vi "Lab Panel V4.88.vi"() -> ()   [LabVIEW 2013] (continued)
              n212 = Bundle(cluster=w241, "Tmp Live"=w237, "Tmp Neut"=w236) -> (w239:T2)  [unwired: 3 in]
              n213 = local write "TEMP LA02"(w243) -> ()
              n214 = local write "SIG LAB02-1"(w239) -> ()
              n215 = local write "SIG LAB02-2"(w238) -> ()
            }
            frame #4 {
              w254 = 0
              n216 = local read "LAB03 TEMP"() -> (w256:T12)
              n217 = Unbundle By Name(w256) -> ("T1 Live"=w249:dbl, "T1 Neut"=w248:dbl, "T2 Live"=w247:dbl, "T2 Neut"=w246:dbl)  [unwired: 2 out]
              n218 = local read "SIG LAB03-1"() -> (w253:T2)
              n219 = local read "SIG LAB03-2"() -> (w252:T2)
              n220 = local read "TEMP LA03"() -> (w257:T9)
              n221 = Bundle By Name(cluster=w257, "TL-1"=w249, "TN-1"=w248, "TL-2"=w247, "TN-2"=w246, "TL -1COUNT"=w254, "TN-1 COUNT"=w254, "TL-2 COUNT"=w254, "TN-2 COUNT"=w254) -> (w255:T9)
              n222 = Bundle(cluster=w252, "Tmp Live"=w247, "Tmp Neut"=w246) -> (w250:T2)  [unwired: 3 in]
              n223 = Bundle(cluster=w253, "Tmp Live"=w249, "Tmp Neut"=w248) -> (w251:T2)  [unwired: 3 in]
              n224 = local write "TEMP LA03"(w255) -> ()
              n225 = local write "SIG LAB03-2"(w250) -> ()
              n226 = local write "SIG LAB03-1"(w251) -> ()
            }
            frame #5 {
              w266 = 0
              n227 = local read "LAB04 TEMP"() -> (w268:T12)
              n228 = Unbundle By Name(w268) -> ("T1 Live"=w261:dbl, "T1 Neut"=w260:dbl, "T2 Live"=w259:dbl, "T2 Neut"=w258:dbl)  [unwired: 2 out]
              n229 = local read "SIG LAB04-2"() -> (w264:T2)
              n230 = local read "SIG LAB04-1"() -> (w265:T2)
              n231 = local read "TEMP LA04"() -> (w269:T9)
              n232 = Bundle By Name(cluster=w269, "TL-1"=w261, "TN-1"=w260, "TL-2"=w259, "TN-2"=w258, "TL -1COUNT"=w266, "TN-1 COUNT"=w266, "TL-2 COUNT"=w266, "TN-2 COUNT"=w266) -> (w267:T9)
              n233 = Bundle(cluster=w264, "Tmp Live"=w259, "Tmp Neut"=w258) -> (w262:T2)  [unwired: 3 in]
              n234 = Bundle(cluster=w265, "Tmp Live"=w261, "Tmp Neut"=w260) -> (w263:T2)  [unwired: 3 in]
              n235 = local write "SIG LAB04-2"(w262) -> ()
              n236 = local write "TEMP LA04"(w267) -> ()
              n237 = local write "SIG LAB04-1"(w263) -> ()
            }
            frame #6 {
              w278 = 0
              n238 = local read "LAB05 TEMP"() -> (w280:T12)
              n239 = Unbundle By Name(w280) -> ("T1 Live"=w273:dbl, "T1 Neut"=w272:dbl, "T2 Live"=w271:dbl, "T2 Neut"=w270:dbl)  [unwired: 2 out]
              n240 = local read "SIG LAB05-2"() -> (w276:T2)
              n241 = local read "SIG LAB05-1"() -> (w277:T2)
              n242 = local read "TEMP LA05"() -> (w281:T9)
              n243 = Bundle By Name(cluster=w281, "TL-1"=w273, "TN-1"=w272, "TL-2"=w271, "TN-2"=w270, "TL -1COUNT"=w278, "TN-1 COUNT"=w278, "TL-2 COUNT"=w278, "TN-2 COUNT"=w278) -> (w279:T9)
              n244 = Bundle(cluster=w276, "Tmp Live"=w271, "Tmp Neut"=w270) -> (w274:T2)  [unwired: 3 in]
              n245 = Bundle(cluster=w277, "Tmp Live"=w273, "Tmp Neut"=w272) -> (w275:T2)  [unwired: 3 in]
              n246 = local write "SIG LAB05-2"(w274) -> ()
              n247 = local write "SIG LAB05-1"(w275) -> ()
              n248 = local write "TEMP LA05"(w279) -> ()
            }
          }
        }
        frame #8 {
          # "enable front panel, all settings done"
          n249 = property on="Tab Control 2" class="TabCtl (strict)"("DisabledEnum"=T16."Enabled" ("Disabled")) -> ()  [unwired: 2 in, 2 out]
          n250 = property on="Tab Control 2" class="TabCtl (strict)"("Value"=0) -> ()  [unwired: 2 in, 2 out]
        }
        frame #9 {
          n251 = property on="Tab Control 2" class="TabCtl (strict)"("Value"=0) -> ()  [unwired: 2 in, 2 out]
        }
      }
    }
    frame #2 {
      n252 = node-c288("loop  delay(mS)") -> (w287:T17)  [unwired: 3 in]
      n253 = timed-loop {
        timing: w287 -> [_]
        timing-out: [_] -> w286
        i -> [w309]
        stop <- "stop" stop-if-true
        n254 = node-c288() -> ()  [unwired: 1 in, 1 out]
        n255 = global write "Global display 1.vi" "stop disp"("stop") -> ()
        n256 = local read "SELECT LAB05-2"() -> (w289:T3)
        n257 = local read "SELECT LAB05-1"() -> (w290:T3)
        n258 = local read "SELECT LAB04-2"() -> (w291:T3)
        n259 = local read "SELECT LAB03-1"() -> (w294:T3)
        n260 = local read "SELECT LAB02-2"() -> (w295:T3)
        n261 = local read "SELECT LAB01-1"() -> (w298:T3)
        n262 = local read "SELECT LAB03-2"() -> (w293:T3)
        n263 = local read "SELECT LAB01-2"() -> (w297:T3)
        n264 = local read "SELECT LAB04-1"() -> (w292:T3)
        n265 = local read "SELECT LAB02-1"() -> (w296:T3)
        n266 = local read "run lab03-2"() -> (w303:bool)
        n267 = local read "run lab04-1"() -> (w302:bool)
        n268 = local read "run lab05-1"() -> (w300:bool)
        n269 = local read "run lab04-2"() -> (w301:bool)
        n270 = local read "run lab05-2"() -> (w299:bool)
        n271 = local read "run lab03-1"() -> (w304:bool)
        n272 = local read "run lab02-2"() -> (w305:bool)
        n273 = local read "run lab02-1"() -> (w306:bool)
        n274 = local read "run lab01-1"() -> (w308:bool)
        n275 = local read "run lab01-2"() -> (w307:bool)
        n276 = stacked-sequence {
          seq-local: [_ w374 _ _ _ _ _ _ _ _ _ _ _ _ _ _ _ _ _ _ _ _ _] -> [_ _ _ _ _ w2474 _ _ _ _ _ _ _ _ _ _ _ _ _ _ _ _ _]
          seq-local: [_ w373 _ _ _ _ _ _ _ _ _ _ _ _ _ _ _ _ _ _ _ _ _] -> [_ _ _ _ _ w2473 _ _ _ _ _ _ _ _ _ _ _ _ _ _ _ _ _]
          seq-local: [_ w360 _ _ _ _ _ _ _ _ _ _ _ _ _ _ _ _ _ _ _ _ _] -> [_ _ _ _ _ w2472 _ _ _ _ _ _ _ _ _ _ _ _ _ _ _ _ _]
          seq-local: [_ w359 _ _ _ _ _ _ _ _ _ _ _ _ _ _ _ _ _ _ _ _ _] -> [_ _ _ _ _ w2471 _ _ _ _ _ _ _ _ _ _ _ _ _ _ _ _ _]
          seq-local: [_ w358 _ _ _ _ _ _ _ _ _ _ _ _ _ _ _ _ _ _ _ _ _] -> [_ _ _ _ _ w2470 _ _ _ _ _ _ _ _ _ _ _ _ _ _ _ _ _]
          seq-local: [_ w357 _ _ _ _ _ _ _ _ _ _ _ _ _ _ _ _ _ _ _ _ _] -> [_ _ _ _ _ w2469 _ _ _ _ _ _ _ _ _ _ _ _ _ _ _ _ _]
          seq-local: [_ w356 _ _ _ _ _ _ _ _ _ _ _ _ _ _ _ _ _ _ _ _ _] -> [_ _ _ _ _ w2468 _ _ _ _ _ _ _ _ _ _ _ _ _ _ _ _ _]
          seq-local: [_ w355 _ _ _ _ _ _ _ _ _ _ _ _ _ _ _ _ _ _ _ _ _] -> [_ _ _ _ _ w2467 _ _ _ _ _ _ _ _ _ _ _ _ _ _ _ _ _]
          seq-local: [_ w354 _ _ _ _ _ _ _ _ _ _ _ _ _ _ _ _ _ _ _ _ _] -> [_ _ _ _ _ w2466 _ _ _ _ _ _ _ _ _ _ _ _ _ _ _ _ _]
          seq-local: [_ w353 _ _ _ _ _ _ _ _ _ _ _ _ _ _ _ _ _ _ _ _ _] -> [_ _ _ _ _ w2465 _ _ _ _ _ _ _ _ _ _ _ _ _ _ _ _ _]
          tunnel: w308 -> [_ _ w390 w637 w2064 w2494 w2809 w3296 _ _ _ _ w3721 _ w4678 _ _ w4965 w5268 w5450 _ _ _]
          tunnel: w307 -> [_ _ w389 w635 w2063 w2493 w2810 w3295 _ _ _ _ w3720 _ w4676 _ _ w4964 w5267 w5448 _ _ _]
          tunnel: w306 -> [_ _ w388 w633 w2062 w2492 w2808 w3294 _ _ _ _ w3719 _ w4674 _ _ w4963 w5266 w5447 _ _ _]
          tunnel: w305 -> [_ _ w387 w631 w2061 w2491 w2807 w3293 _ _ _ _ w3718 _ w4672 _ _ w4962 w5265 w5446 _ _ _]
          tunnel: w304 -> [_ _ w386 w629 w2060 w2490 w2806 w3292 _ _ _ _ w3717 _ w4670 _ _ w4961 w5264 w5445 _ _ _]
          tunnel: w303 -> [_ _ w385 w627 w2059 w2489 w2805 w3291 _ _ _ _ w3716 _ w4668 _ _ w4960 w5263 w5444 _ _ _]
          tunnel: w302 -> [_ _ w384 w625 w2058 w2488 w2804 w3290 _ _ _ _ w3715 _ w4666 _ _ w4959 w5262 w5443 _ _ _]
          tunnel: w301 -> [_ _ w383 w623 w2057 w2487 w2803 w3289 _ _ _ _ w3714 _ w4664 _ _ w4958 w5261 w5442 _ _ _]
          tunnel: w300 -> [_ _ w382 w621 w2056 w2486 w2802 w3288 _ _ _ _ w3713 _ w4662 _ _ w4957 w5260 w5441 _ _ _]
          tunnel: w299 -> [_ _ w381 w619 w2055 w2485 w2801 w3287 _ _ _ _ w3712 _ w4660 _ _ w4956 w5259 w5440 _ _ _]
          tunnel: w298 -> [_ _ _ w636 w2054 w2484 _ _ _ _ _ _ _ _ w4680 _ _ _ _ _ w5788 _ _]
          tunnel: w297 -> [_ _ _ w634 w2053 w2483 _ _ _ _ _ _ _ _ w4675 _ _ _ _ _ w5787 _ _]
          tunnel: w296 -> [_ _ _ w632 w2052 w2482 _ _ _ _ _ _ _ _ w4673 _ _ _ _ _ w5786 _ _]
          tunnel: w295 -> [_ _ _ w630 w2051 w2481 _ _ _ _ _ _ _ _ w4671 _ _ _ _ _ w5785 _ _]
          tunnel: w294 -> [_ _ _ w628 w2050 w2480 _ _ _ _ _ _ _ _ w4669 _ _ _ _ _ w5784 _ _]
          tunnel: w293 -> [_ _ _ w626 w2049 w2479 _ _ _ _ _ _ _ _ w4667 _ _ _ _ _ w5783 _ _]
          tunnel: w292 -> [_ _ _ w624 w2048 w2478 _ _ _ _ _ _ _ _ w4665 _ _ _ _ _ w5782 _ _]
          tunnel: w291 -> [_ _ _ w622 w2047 w2477 _ _ _ _ _ _ _ _ w4663 _ _ _ _ _ w5781 _ _]
          tunnel: w290 -> [_ _ _ w620 w2046 w2476 _ _ _ _ _ _ _ _ w4661 _ _ _ _ _ w5780 _ _]
          tunnel: w289 -> [_ _ _ w618 w2045 w2475 _ _ _ _ _ _ _ _ w4659 _ _ _ _ _ w5779 _ _]
          frame #0 {
            w316 = FALSE
            w321 = 0.5
            # "set up cycle control"
            n277 = local read "jig cycle"() -> (w320:dbl)
            n278 = local read "Amps Fail level"() -> (w314:dbl)
            n279 = Divide(x="JIG ON TIME (S)", y=w321) -> (x/y=→"on loops":dbl)
            n280 = Divide(x="JIG OFF TIME (S)", y=w321) -> (x/y=→"off loops":dbl)
            n281 = global write "Global display 3.vi" "Amps Fail"(w314) -> ()
            n282 = Increment(x=w320) -> (x+1=w319:dbl)
            n283 = local write "TEMP"(w316) -> ()
            n284 = local write "AI"(w316) -> ()
            n285 = local read "Network Directory"() -> (w313:path)
            n286 = local write "jig cycle"(w319) -> ()
            n287 = call "sub vi - check network dir v2.vi"("PATH"=w313) -> ("error"=w312:bool)  [unwired: 10 in]
            n288 = local write "network error"(w312) -> ()
            n289 = global write "Global display 3.vi" "network drive"(w312) -> ()
            n290 = event shown="[1] \"ADMIN\": Value Change" {
              selector: _ -> [_ _]
              dyn-events: _ -> [_ _]
              timeout: 10 -> [_ _]
              event Timeout {
                n291 = event-data() -> ()  [unwired: 1 in, 3 out]
              }
              event "ADMIN": Value Change {
                n292 = event-data() -> ()  [unwired: 1 in, 6 out]
                n293 = stacked-sequence {
                  seq-local: [_ w325 _] -> [_ _ w326]
                  frame #0 {
                    n294 = global write "Global 1.vi" "password"("9949") -> ()
                  }
                  frame #1 {
                    n295 = call "sub vi - password 1.vi"() -> ("RESULT"=w325:bool)  [unwired: 11 in]
                  }
                  frame #2 {
                    w328 = FALSE
                    n296 = property on="Tab Control 2" class="TabCtl (strict)"() -> ("Pages"=w332:refnum<vi>[])  [unwired: 2 in, 2 out]
                    n297 = Select(t=TRUE, s=w326, f=w328) -> (s? t:f=w327:bool)
                    n298 = Index Array(array=w332, index=8) -> (element=w330:refnum<vi>)
                    n299 = property class="Page"(reference=w330, "PageVis"=w327) -> ()  [unwired: 1 in, 2 out]
                    n300 = local write "ADMIN"(w328) -> ()
                  }
                }
              }
            }
          }
          frame #1 {
            w370 = 60.0
            # "convert temperature rise minutes to cycles"
            n301 = local read "SET LAB05-2"() -> (w334:T5)
            n302 = local read "SET LAB05-1"() -> (w336:T5)
            n303 = local read "SET LAB04-2"() -> (w338:T5)
            n304 = local read "SET LAB01-1"() -> (w352:T5)
            n305 = local read "SET LAB01-2"() -> (w350:T5)
            n306 = local read "SET LAB02-2"() -> (w346:T5)
            n307 = local read "SET LAB04-1"() -> (w340:T5)
            n308 = local read "SET LAB03-1"() -> (w344:T5)
            n309 = local read "SET LAB03-2"() -> (w342:T5)
            n310 = local read "SET LAB02-1"() -> (w348:T5)
            n311 = local read "JIG OFF TIME (S)"() -> (w375:dbl)
            n312 = local read "JIG ON TIME (S)"() -> (w376:dbl)
            n313 = Unbundle(w334) -> ("T-RISE mins"=w333:dbl)  [unwired: 4 out]
            n314 = Unbundle(w336) -> ("T-RISE mins"=w335:dbl)  [unwired: 4 out]
            n315 = Unbundle(w352) -> ("T-RISE mins"=w351:dbl)  [unwired: 4 out]
            n316 = Unbundle(w338) -> ("T-RISE mins"=w337:dbl)  [unwired: 4 out]
            n317 = Unbundle(w350) -> ("T-RISE mins"=w349:dbl)  [unwired: 4 out]
            n318 = Unbundle(w348) -> ("T-RISE mins"=w347:dbl)  [unwired: 4 out]
            n319 = Unbundle(w340) -> ("T-RISE mins"=w339:dbl)  [unwired: 4 out]
            n320 = Unbundle(w346) -> ("T-RISE mins"=w345:dbl)  [unwired: 4 out]
            n321 = Unbundle(w342) -> ("T-RISE mins"=w341:dbl)  [unwired: 4 out]
            n322 = Unbundle(w344) -> ("T-RISE mins"=w343:dbl)  [unwired: 4 out]
            n323 = Add(x=w376, y=w375) -> (x+y=w369:dbl)
            n324 = Multiply(x=w370, y=w341) -> (x*y=w365:dbl)
            n325 = Multiply(x=w370, y=w339) -> (x*y=w364:dbl)
            n326 = Multiply(x=w370, y=w337) -> (x*y=w363:dbl)
            n327 = Multiply(x=w370, y=w335) -> (x*y=w362:dbl)
            n328 = Multiply(x=w370, y=w333) -> (x*y=w361:dbl)
            n329 = Multiply(x=w370, y=w349) -> (x*y=w371:dbl)
            n330 = Multiply(x=w370, y=w343) -> (x*y=w366:dbl)
            n331 = Multiply(x=w370, y=w351) -> (x*y=w372:dbl)
            n332 = Multiply(x=w370, y=w347) -> (x*y=w368:dbl)
            n333 = Multiply(x=w370, y=w345) -> (x*y=w367:dbl)
            n334 = Divide(x=w362, y=w369) -> (x/y=w354:dbl)
            n335 = Divide(x=w363, y=w369) -> (x/y=w355:dbl)
            n336 = Divide(x=w364, y=w369) -> (x/y=w356:dbl)
            n337 = Divide(x=w361, y=w369) -> (x/y=w353:dbl)
            n338 = Divide(x=w366, y=w369) -> (x/y=w358:dbl)
            n339 = Divide(x=w372, y=w369) -> (x/y=w374:dbl)
            n340 = Divide(x=w371, y=w369) -> (x/y=w373:dbl)
            n341 = Divide(x=w368, y=w369) -> (x/y=w360:dbl)
            n342 = Divide(x=w367, y=w369) -> (x/y=w359:dbl)
            n343 = Divide(x=w365, y=w369) -> (x/y=w357:dbl)
          }
          frame #2 {
            # "control cycle loops"
            n344 = local read "JIG OFF TIME (S)"() -> (w379:dbl)
            n345 = local read "JIG ON TIME (S)"() -> (w378:dbl)
            n346 = local read "jig cycle"() -> (w392:dbl)
            n347 = local read "on loops"() -> (w394:dbl)
            n348 = local read "off loops"() -> (w393:dbl)
            n349 = Add(x=w379, y=w378) -> (x+y=w377:dbl)
            n350 = Add(x=w394, y=w393) -> (x+y=w380:dbl)
            n351 = Greater Or Equal?(x=w392, y=w380) -> (x >= y?=w391:bool)
            n352 = case shown="True" w391 {
              tunnel: w390 -> [_ w427]
              tunnel: w389 -> [_ w426]
              tunnel: w388 -> [_ w425]
              tunnel: w387 -> [_ w424]
              tunnel: w386 -> [_ w423]
              tunnel: w385 -> [_ w422]
              tunnel: w384 -> [_ w421]
              tunnel: w383 -> [_ w420]
              tunnel: w382 -> [_ w419]
              tunnel: w381 -> [_ w418]
              tunnel: w377 -> [_ w417]
              frame False {
              }
              frame True {
                # "increment cycle value and convert cycles to minutes for temp rise"
                n353 = stacked-sequence {
                  frame #0 {
                    n354 = local read "PANEL #"() -> (w430:dbl)
                    n355 = Increment(x=w430) -> (x+1=w429:dbl)
                    n356 = local write "PANEL #"(w429) -> ()
                  }
                  frame #1 {
                    n357 = local read "PANEL #"() -> (w431:dbl)
                    n358 = Greater?(x=w431, y=5) -> (0:w433:bool)
                    n359 = case shown="True" w433 {
                      frame False {
                      }
                      frame True {
                        n360 = local write "PANEL #"(1) -> ()
                      }
                    }
                  }
                }
                n361 = local read "JIG RELAY CYCLES"() -> (w416:T8)
                n362 = Unbundle By Name(w416) -> ("LAB01-1"=w414:dbl, "LAB01-2"=w412:dbl, "LAB02-1"=w410:dbl, "LAB02-2"=w408:dbl, "LAB03-1"=w406:dbl, "LAB03-2"=w404:dbl, "LAB04-1"=w402:dbl, "LAB04-2"=w400:dbl, "LAB05-1"=w398:dbl, "LAB05-2"=w396:dbl)
                n363 = stacked-sequence {
                  tunnel: w427 -> [w445 _ _ _ _ _ _ _ _ _]
                  tunnel: w426 -> [_ w462 _ _ _ _ _ _ _ _]
                  tunnel: w425 -> [_ _ w479 _ _ _ _ _ _ _]
                  tunnel: w424 -> [_ _ _ w496 _ _ _ _ _ _]
                  tunnel: w423 -> [_ _ _ _ w513 _ _ _ _ _]
                  tunnel: w422 -> [_ _ _ _ _ w530 _ _ _ _]
                  tunnel: w421 -> [_ _ _ _ _ _ w547 _ _ _]
                  tunnel: w420 -> [_ _ _ _ _ _ _ w564 _ _]
                  tunnel: w419 -> [_ _ _ _ _ _ _ _ w581 _]
                  tunnel: w418 -> [_ _ _ _ _ _ _ _ _ w598]
                  tunnel: w417 -> [w442 w459 w476 w493 w510 w527 w544 w561 w578 w595]
                  tunnel: w414 -> [w436 _ _ _ _ _ _ _ _ _]
                  tunnel: [w435 _ _ _ _ _ _ _ _ _] -> w413
                  tunnel: w412 -> [_ w453 _ _ _ _ _ _ _ _]
                  tunnel: [_ w452 _ _ _ _ _ _ _ _] -> w411
                  tunnel: w410 -> [_ _ w470 _ _ _ _ _ _ _]
                  tunnel: [_ _ w469 _ _ _ _ _ _ _] -> w409
                  tunnel: w408 -> [_ _ _ w487 _ _ _ _ _ _]
                  tunnel: [_ _ _ w486 _ _ _ _ _ _] -> w407
                  tunnel: w406 -> [_ _ _ _ w504 _ _ _ _ _]
                  tunnel: [_ _ _ _ w503 _ _ _ _ _] -> w405
                  tunnel: w404 -> [_ _ _ _ _ w521 _ _ _ _]
                  tunnel: [_ _ _ _ _ w520 _ _ _ _] -> w403
                  tunnel: w402 -> [_ _ _ _ _ _ w538 _ _ _]
                  tunnel: [_ _ _ _ _ _ w537 _ _ _] -> w401
                  tunnel: w400 -> [_ _ _ _ _ _ _ w555 _ _]
                  tunnel: [_ _ _ _ _ _ _ w554 _ _] -> w399
                  tunnel: w398 -> [_ _ _ _ _ _ _ _ w572 _]
                  tunnel: [_ _ _ _ _ _ _ _ w571 _] -> w397
                  tunnel: w396 -> [_ _ _ _ _ _ _ _ _ w589]
                  tunnel: [_ _ _ _ _ _ _ _ _ w588] -> w395
                  frame #0 {
                    n364 = local read "DISP LAB01-1"() -> (w440:T4)
                    n365 = Unbundle(w440) -> ("CYCLE"=w441:dbl)  [unwired: 2 out]
                    n366 = case shown="True" w445 {
                      tunnel: w441 -> [w447 w451]
                      tunnel: [w447 w450] -> w439
                      tunnel: w436 -> [w446 w449]
                      tunnel: [w446 w448] -> w435
                      frame False {
                      }
                      frame True {
                        n367 = Increment(x=w449) -> (x+1=w448:dbl)
                        n368 = Increment(x=w451) -> (x+1=w450:dbl)
                      }
                    }
                    n369 = Multiply(x=w439, y=w442) -> (x*y=w443:dbl)
                    n370 = Divide(x=w443, y=60.0) -> (x/y=w438:dbl)
                    n371 = Bundle(cluster=w440, "CYCLE"=w439, "MINS"=w438) -> (w437:T4)  [unwired: 1 in]
                    n372 = local write "DISP LAB01-1"(w437) -> ()
                  }
                  frame #1 {
                    n373 = local read "DISP LAB01-2"() -> (w457:T4)
                    n374 = Unbundle(w457) -> ("CYCLE"=w458:dbl)  [unwired: 2 out]
                    n375 = case shown="True" w462 {
                      tunnel: w458 -> [w464 w468]
                      tunnel: [w464 w467] -> w455
                      tunnel: w453 -> [w463 w466]
                      tunnel: [w463 w465] -> w452
                      frame False {
                      }
                      frame True {
                        n376 = Increment(x=w466) -> (x+1=w465:dbl)
                        n377 = Increment(x=w468) -> (x+1=w467:dbl)
                      }
                    }
                    n378 = Multiply(x=w455, y=w459) -> (x*y=w460:dbl)
                    n379 = Divide(x=w460, y=60.0) -> (x/y=w454:dbl)
                    n380 = Bundle(cluster=w457, "CYCLE"=w455, "MINS"=w454) -> (w456:T4)  [unwired: 1 in]
                    n381 = local write "DISP LAB01-2"(w456) -> ()
                  }
                  frame #2 {
                    n382 = local read "DISP LAB02-1"() -> (w474:T4)
                    n383 = Unbundle(w474) -> ("CYCLE"=w475:dbl)  [unwired: 2 out]
                    n384 = case shown="True" w479 {
                      tunnel: [w481 w485] -> w472
                      tunnel: w475 -> [w481 w484]
                      tunnel: w470 -> [w480 w483]
                      tunnel: [w480 w482] -> w469
                      frame False {
                      }
                      frame True {
                        n385 = Increment(x=w483) -> (x+1=w482:dbl)
                        n386 = Increment(x=w484) -> (x+1=w485:dbl)
                      }
                    }
                    n387 = Multiply(x=w472, y=w476) -> (x*y=w477:dbl)
                    n388 = Divide(x=w477, y=60.0) -> (x/y=w471:dbl)
                    n389 = Bundle(cluster=w474, "CYCLE"=w472, "MINS"=w471) -> (w473:T4)  [unwired: 1 in]
                    n390 = local write "DISP LAB02-1"(w473) -> ()
                  }
                  frame #3 {
                    n391 = local read "DISP LAB02-2"() -> (w491:T4)
                    n392 = Unbundle(w491) -> ("CYCLE"=w492:dbl)  [unwired: 2 out]
                    n393 = case shown="True" w496 {
                      tunnel: [w498 w502] -> w490
                      tunnel: w492 -> [w498 w501]
                      tunnel: w487 -> [w497 w500]
                      tunnel: [w497 w499] -> w486
                      frame False {
                      }
                      frame True {
                        n394 = Increment(x=w500) -> (x+1=w499:dbl)
                        n395 = Increment(x=w501) -> (x+1=w502:dbl)
                      }
                    }
                    n396 = Multiply(x=w490, y=w493) -> (x*y=w494:dbl)
                    n397 = Divide(x=w494, y=60.0) -> (x/y=w489:dbl)
                    n398 = Bundle(cluster=w491, "CYCLE"=w490, "MINS"=w489) -> (w488:T4)  [unwired: 1 in]
                    n399 = local write "DISP LAB02-2"(w488) -> ()
                  }
                  frame #4 {
                    n400 = local read "DISP LAB03-1"() -> (w508:T4)
                    n401 = Unbundle(w508) -> ("CYCLE"=w509:dbl)  [unwired: 2 out]
                    n402 = case shown="True" w513 {
                      tunnel: [w515 w519] -> w505
                      tunnel: w509 -> [w515 w518]
                      tunnel: w504 -> [w514 w517]
                      tunnel: [w514 w516] -> w503
                      frame False {
                      }
                      frame True {
                        n403 = Increment(x=w517) -> (x+1=w516:dbl)
                        n404 = Increment(x=w518) -> (x+1=w519:dbl)
                      }
                    }
                    n405 = Multiply(x=w505, y=w510) -> (x*y=w511:dbl)
                    n406 = Divide(x=w511, y=60.0) -> (x/y=w506:dbl)
                    n407 = Bundle(cluster=w508, "CYCLE"=w505, "MINS"=w506) -> (w507:T4)  [unwired: 1 in]
                    n408 = local write "DISP LAB03-1"(w507) -> ()
                  }
                  frame #5 {
                    n409 = local read "DISP LAB03-2"() -> (w525:T4)
                    n410 = Unbundle(w525) -> ("CYCLE"=w526:dbl)  [unwired: 2 out]
                    n411 = case shown="True" w530 {
                      tunnel: [w532 w536] -> w524
                      tunnel: w526 -> [w532 w535]
                      tunnel: w521 -> [w531 w534]
                      tunnel: [w531 w533] -> w520
                      frame False {
                      }
                      frame True {
                        n412 = Increment(x=w534) -> (x+1=w533:dbl)
                        n413 = Increment(x=w535) -> (x+1=w536:dbl)
                      }
                    }
                    n414 = Multiply(x=w524, y=w527) -> (x*y=w528:dbl)
                    n415 = Divide(x=w528, y=60.0) -> (x/y=w523:dbl)
                    n416 = Bundle(cluster=w525, "CYCLE"=w524, "MINS"=w523) -> (w522:T4)  [unwired: 1 in]
                    n417 = local write "DISP LAB03-2"(w522) -> ()
                  }
                  frame #6 {
                    n418 = local read "DISP LAB04-1"() -> (w542:T4)
                    n419 = Unbundle(w542) -> ("CYCLE"=w543:dbl)  [unwired: 2 out]
                    n420 = case shown="True" w547 {
                      tunnel: [w549 w553] -> w540
                      tunnel: w543 -> [w549 w552]
                      tunnel: w538 -> [w548 w551]
                      tunnel: [w548 w550] -> w537
                      frame False {
                      }
                      frame True {
                        n421 = Increment(x=w551) -> (x+1=w550:dbl)
                        n422 = Increment(x=w552) -> (x+1=w553:dbl)
                      }
                    }
                    n423 = Multiply(x=w540, y=w544) -> (x*y=w545:dbl)
                    n424 = Divide(x=w545, y=60.0) -> (x/y=w539:dbl)
                    n425 = Bundle(cluster=w542, "CYCLE"=w540, "MINS"=w539) -> (w541:T4)  [unwired: 1 in]
                    n426 = local write "DISP LAB04-1"(w541) -> ()
                  }
                  frame #7 {
                    n427 = local read "DISP LAB04-2"() -> (w559:T4)
                    n428 = Unbundle(w559) -> ("CYCLE"=w560:dbl)  [unwired: 2 out]
                    n429 = case shown="True" w564 {
                      tunnel: [w566 w570] -> w557
                      tunnel: w560 -> [w566 w569]
                      tunnel: w555 -> [w565 w568]
                      tunnel: [w565 w567] -> w554
                      frame False {
                      }
                      frame True {
                        n430 = Increment(x=w568) -> (x+1=w567:dbl)
                        n431 = Increment(x=w569) -> (x+1=w570:dbl)
                      }
                    }
                    n432 = Multiply(x=w557, y=w561) -> (x*y=w563:dbl)
                    n433 = Divide(x=w563, y=60.0) -> (x/y=w556:dbl)
                    n434 = Bundle(cluster=w559, "CYCLE"=w557, "MINS"=w556) -> (w558:T4)  [unwired: 1 in]
                    n435 = local write "DISP LAB04-2"(w558) -> ()
                  }
                  frame #8 {
                    n436 = local read "DISP LAB05-1"() -> (w576:T4)
                    n437 = Unbundle(w576) -> ("CYCLE"=w577:dbl)  [unwired: 2 out]
                    n438 = case shown="True" w581 {
                      tunnel: [w583 w587] -> w574
                      tunnel: w577 -> [w583 w586]
                      tunnel: w572 -> [w582 w585]
                      tunnel: [w582 w584] -> w571
                      frame False {
                      }
                      frame True {
                        n439 = Increment(x=w585) -> (x+1=w584:dbl)
                        n440 = Increment(x=w586) -> (x+1=w587:dbl)
                      }
                    }
                    n441 = Multiply(x=w574, y=w578) -> (x*y=w579:dbl)
                    n442 = Divide(x=w579, y=60.0) -> (x/y=w573:dbl)
                    n443 = Bundle(cluster=w576, "CYCLE"=w574, "MINS"=w573) -> (w575:T4)  [unwired: 1 in]
                    n444 = local write "DISP LAB05-1"(w575) -> ()
                  }
                  frame #9 {
                    n445 = local read "DISP LAB05-2"() -> (w594:T4)
                    n446 = Unbundle(w594) -> ("CYCLE"=w593:dbl)  [unwired: 2 out]
                    n447 = case shown="True" w598 {
                      tunnel: [w600 w604] -> w592
                      tunnel: w593 -> [w600 w603]
                      tunnel: w589 -> [w599 w602]
                      tunnel: [w599 w601] -> w588
                      frame False {
                      }
                      frame True {
                        n448 = Increment(x=w602) -> (x+1=w601:dbl)
                        n449 = Increment(x=w603) -> (x+1=w604:dbl)
                      }
                    }
                    n450 = Multiply(x=w592, y=w595) -> (x*y=w596:dbl)
                    n451 = Divide(x=w596, y=60.0) -> (x/y=w591:dbl)
                    n452 = Bundle(cluster=w594, "CYCLE"=w592, "MINS"=w591) -> (w590:T4)  [unwired: 1 in]
                    n453 = local write "DISP LAB05-2"(w590) -> ()
                  }
                }
                n454 = local write "jig cycle"(0) -> ()
                n455 = Bundle By Name(cluster=w416, "LAB01-1"=w413, "LAB01-2"=w411, "LAB02-1"=w409, "LAB02-2"=w407, "LAB03-1"=w405, "LAB03-2"=w403, "LAB04-1"=w401, "LAB04-2"=w399, "LAB05-1"=w397, "LAB05-2"=w395) -> (w415:T8)
                n456 = local write "JIG RELAY CYCLES"(w415) -> ()
              }
            }
          }
          frame #3 {
            # "START & STOP test RUN switch change, start test if true and stop test if false"
            n457 = Get Date/Time In Seconds() -> (seconds since 1Jan1904=w616:timestamp)
            n458 = local read "C drive data root dir"() -> (w609:path)
            n459 = Format Date/Time String(time format string (%c)="%b\\%a%d", seconds (now)=w616) -> (date/time string=w640:string)  [unwired: 1 in]
            n460 = Format Date/Time String(time format string (%c)="%H%M", seconds (now)=w616) -> (date/time string=w638:string)  [unwired: 1 in]
            n461 = Format Date/Time String(time format string (%c)="LabPanel%Y", seconds (now)=w616) -> (date/time string=w615:string)  [unwired: 1 in]
            n462 = Path To String(path=w609) -> (string=w612:string)
            n463 = global write "Global 1.vi" "C drive root path"(w609) -> ()
            n464 = local read "Ref deg C"() -> (w605:dbl)
            n465 = Concatenate Strings(w612, "\\") -> (w610:string)
            n466 = event shown="[1] \"RUN LAB01-1\": Value Change" {
              selector: _ -> [_ _ _ _ _ _ _ _ _ _ _]
              dyn-events: _ -> [_ _ _ _ _ _ _ _ _ _ _]
              timeout: 10 -> [_ _ _ _ _ _ _ _ _ _ _]
              tunnel: w610 -> [_ w653 w793 w934 w1074 w1214 w1354 w1494 w1634 w1774 w1915]
              tunnel: w640 -> [_ w652 w792 w933 w1073 w1213 w1353 w1493 w1633 w1773 w1914]
              tunnel: w638 -> [_ w650 w791 w932 w1072 w1212 w1352 w1492 w1632 w1772 w1913]
              tunnel: w636 -> [_ w651 _ _ _ _ _ _ _ _ _]
              tunnel: w637 -> [_ _ _ _ _ _ _ _ _ _ _]
              tunnel: w635 -> [_ _ _ _ _ _ _ _ _ _ _]
              tunnel: w634 -> [_ _ w790 _ _ _ _ _ _ _ _]
              tunnel: w633 -> [_ _ _ _ _ _ _ _ _ _ _]
              tunnel: w632 -> [_ _ _ w931 _ _ _ _ _ _ _]
              tunnel: w631 -> [_ _ _ _ _ _ _ _ _ _ _]
              tunnel: w630 -> [_ _ _ _ w1071 _ _ _ _ _ _]
              tunnel: w629 -> [_ _ _ _ _ _ _ _ _ _ _]
              tunnel: w628 -> [_ _ _ _ _ w1211 _ _ _ _ _]
              tunnel: w627 -> [_ _ _ _ _ _ _ _ _ _ _]
              tunnel: w626 -> [_ _ _ _ _ _ w1351 _ _ _ _]
              tunnel: w625 -> [_ _ _ _ _ _ _ _ _ _ _]
              tunnel: w624 -> [_ _ _ _ _ _ _ w1491 _ _ _]
              tunnel: w623 -> [_ _ _ _ _ _ _ _ _ _ _]
              tunnel: w622 -> [_ _ _ _ _ _ _ _ w1631 _ _]
              tunnel: w621 -> [_ _ _ _ _ _ _ _ _ _ _]
              tunnel: w620 -> [_ _ _ _ _ _ _ _ _ w1771 _]
              tunnel: w619 -> [_ _ _ _ _ _ _ _ _ _ _]
              tunnel: w618 -> [_ _ _ _ _ _ _ _ _ _ w1912]
              tunnel: w615 -> [_ w649 w789 w930 w1070 w1210 w1350 w1490 w1630 w1770 w1911]
              tunnel: [_ w648 w788 w929 w1069 w1209 w1349 w1489 w1629 w1769 w1910] -> w613
              tunnel: "RESET CYCLES TO ZERO?" -> [_ w647 w786 w927 w1067 w1207 w1347 w1487 w1627 w1767 w1908]
              tunnel: "YES" -> [_ w646 w785 w926 w1066 w1206 w1346 w1486 w1626 w1766 w1907]
              tunnel: "NO" -> [_ w645 w784 w925 w1065 w1205 w1345 w1485 w1625 w1765 w1906]
              tunnel: w605 -> [_ w642 w783 w923 w1064 w1204 w1344 w1484 w1624 w1764 w1904]
              event Timeout {
                n467 = event-data() -> ()  [unwired: 1 in, 3 out]
              }
              event "RUN LAB01-1": Value Change {
                n468 = event-data() -> ("NewVal"=w643:bool)  [unwired: 1 in, 5 out]
                n469 = local read "SIG LAB01-1"() -> (w644:T2)
                n470 = local write "run lab01-1"(w643) -> ()
                n471 = case shown="True" w643 {
                  tunnel: w653 -> [_ w691]
                  tunnel: w652 -> [_ w690]
                  tunnel: w651 -> [w655 w689]
                  tunnel: w650 -> [_ w688]
                  tunnel: w649 -> [_ w687]
                  tunnel: [w654 w686] -> w648
                  tunnel: w647 -> [_ w685]
                  tunnel: w646 -> [_ w684]
                  tunnel: w645 -> [_ w683]
                  tunnel: w644 -> [_ w682]
                  tunnel: w642 -> [_ w681]
                  frame False {
                    # "stop test"
                    n472 = stacked-sequence {
                      tunnel: w655 -> [_ w667 _]
                      tunnel: [_ w659 _] -> w654
                      frame #0 {
                        n473 = local read "DISP LAB01-1"() -> (w658:T4)
                        n474 = Bundle(cluster=w658, "STATUS"="STOP") -> (w656:T4)  [unwired: 2 in]
                        n475 = local write "DISP LAB01-1"(w656) -> ()
                      }
                      frame #1 {
                        n476 = local read "DISP LAB01-1"() -> (w666:T4)
                        n477 = Unbundle(w666) -> ("CYCLE"=w664:dbl, "MINS"=w665:dbl)  [unwired: 1 out]
                        n478 = case shown="\"CYCLE TEST\"" w667 {
                          tunnel: w665 -> [_ _ w674]
                          tunnel: w664 -> [w672 w673 _]
                          tunnel: [w672 w673 w674] -> w663
                          frame "CHART TEST", Default {
                          }
                          frame "CYCLE TEST" {
                          }
                          frame "T-RISE TEST" {
                          }
                        }
                        n479 = local read "TDMS LAB01-1"() -> (w671:refnum<k34>)
                        n480 = Build Array("STOPPED") -> (w668:string[])
                        n481 = Build Array(w663) -> (w662:dbl[])
                        n482 = TDMS Write(0:w671, 5:"TEST RESULT", 7:w668, 9:w662) -> (4:w660:refnum<k34>, 15:w661:errorcluster)  [unwired: 2 in, 2 out]
                        n483 = TDMS Close(8:w661, 11:w660) -> (0:w659:errorcluster)  [unwired: 1 out]
                      }
                      frame #2 {
                        n484 = stacked-sequence {
                          tunnel: "LAB01-1" -> [w677 w679]
                          frame #0 {
                            n485 = call "sub vi - defrag tdms v1.vi"("panel id"=w677) -> ("error out"=w676:errorcluster)  [unwired: 10 in]
                            n486 = local write "data file error"(w676) -> ()
                          }
                          frame #1 {
                            n487 = call "Save data file (stop) v3.vi"("panel id"=w679) -> ("network file save error"=w678:errorcluster)  [unwired: 9 in, 1 out]
                            n488 = local write "RESULT LAB01-1"(FALSE) -> ()
                            n489 = local write "data file error"(w678) -> ()
                          }
                        }
                      }
                    }
                  }
                  frame True {
                    n490 = stacked-sequence {
                      seq-local: [w693 _] -> [_ w697]
                      tunnel: w691 -> [_ w707]
                      tunnel: w690 -> [_ w706]
                      tunnel: w689 -> [_ w705]
                      tunnel: w688 -> [_ w704]
                      tunnel: w687 -> [_ w703]
                      tunnel: [_ w702] -> w686
                      tunnel: w685 -> [_ w701]
                      tunnel: w684 -> [_ w700]
                      tunnel: w683 -> [_ w699]
                      tunnel: w682 -> [w695 w698]
                      tunnel: w681 -> [_ w696]
                      frame #0 {
                        n491 = Unbundle(w695) -> ("AMPS"=w694:dbl)  [unwired: 4 out]
                        n492 = call "Check For Amps on v1.vi"("ID"="LAB01-1", "amps"=w694) -> ("amps"=w693:bool)  [unwired: 9 in]
                      }
                      frame #1 {
                        n493 = case shown="True" w697 {
                          tunnel: w707 -> [_ w720]
                          tunnel: w706 -> [_ w719]
                          tunnel: w705 -> [_ w718]
                          tunnel: w704 -> [_ w717]
                          tunnel: w703 -> [_ w716]
                          tunnel: [errorcluster {"status"=FALSE, "code"=0, "source"=""} ("error out") w715] -> w702
                          tunnel: w701 -> [_ w714]
                          tunnel: w700 -> [_ w713]
                          tunnel: w699 -> [_ w712]
                          tunnel: w698 -> [_ w711]
                          tunnel: w696 -> [_ w710]
                          frame False {
                            w708 = FALSE
                            n494 = local write "RUN LAB01-1"(w708) -> ()
                            n495 = local write "run lab01-1"(w708) -> ()
                          }
                          frame True {
                            n496 = stacked-sequence {
                              seq-local: [w721 _ _ _ _] -> [_ w742 _ _ _]
                              tunnel: w720 -> [w726 _ _ _ _]
                              tunnel: w719 -> [w722 _ _ _ _]
                              tunnel: w718 -> [w736 _ _ _ _]
                              tunnel: w717 -> [w729 _ _ _ _]
                              tunnel: w716 -> [w724 _ _ _ _]
                              tunnel: [_ w743 _ _ _] -> w715
                              tunnel: w714 -> [_ _ _ w764 _]
                              tunnel: w713 -> [_ _ _ w774 _]
                              tunnel: w712 -> [_ _ _ w773 _]
                              tunnel: w711 -> [_ _ _ _ _]
                              tunnel: w710 -> [_ _ _ _ w780]
                              frame #0 {
                                w723 = "\\"
                                n497 = case shown="\"CHART TEST\", Default" w736 {
                                tunnel: ["L01-1-CHART TEST-" "L01-1-CYCLE TEST-" "L01-1-T-RISE TEST-"] -> w732
                                frame "CHART TEST", Default {
                                }
                                frame "CYCLE TEST" {
                                }
                                frame "T-RISE TEST" {
                                }
                                }
                                n498 = local read "SET LAB01-1"() -> (w731:T5)
                                n499 = Unbundle(w731) -> ("DESCRIPTION"=w730:string)  [unwired: 4 out]
                                n500 = Concatenate Strings(w726, "\\", w724, w723, w722, w723) -> (w733:string)
                                n501 = String To Path(string=w733) -> (path=w735:path)
                                n502 = Concatenate Strings(w733, w732, w730, "-", w729, ".tdms") -> (w721:string)
                                n503 = Create Folder(path (use dialog)=w735) -> (error out=w734:errorcluster)  [unwired: 2 in, 2 out]
                                n504 = call <vilib>:"Clear Errors.vi"("error in (no error)"=w734) -> ()  [unwired: 6 in, 1 out]
                                n505 = global write "Global 1.vi" "LAB01-1 FILE"(w721) -> ()
                              }
                              frame #1 {
                                (unwired) FALSE
                                n506 = String To Path(string=w742) -> (path=w740:path)
                                n507 = TDMS Open(6:FALSE, 10:T20."create or replace" ("operation (0:open)"), 11:w740) -> (0:w743:errorcluster, 3:→"TDMS LAB01-1":refnum<k34>)  [unwired: 4 in]
                              }
                              frame #2 {
                                n508 = local read "TDMS LAB01-1"() -> (w762:refnum<k34>)
                                n509 = local read "SET LAB01-1"() -> (w751:T5)
                                n510 = Build Array("Testers Name", "Description", "Set Test Cycles", "T-Rise minutes", "T-Rise Deg C") -> (w752:string[])
                                n511 = Unbundle(w751) -> ("NAME"=w750:string, "DESCRIPTION"=w749:string, "CYCLES"=w748:dbl, "T-RISE mins"=w747:dbl, "T-RISE deg C"=w746:dbl)
                                n512 = Number To Decimal String(number=w748) -> (decimal integer string=w761:string)  [unwired: 1 in]
                                n513 = Number To Decimal String(number=w747) -> (decimal integer string=w760:string)  [unwired: 1 in]
                                n514 = Number To Decimal String(number=w746) -> (decimal integer string=w759:string)  [unwired: 1 in]
                                n515 = Build Array(w750, w749, w761, w760, w759) -> (w758:string[])
                                n516 = TDMS Set Properties(5:w758, 7:w752, 11:w762) -> ()  [unwired: 3 in, 4 out]
                              }
                              frame #3 {
                                n517 = local read "DISP LAB01-1"() -> (w772:T4)
                                n518 = Concatenate Strings("LAB01-1  ", w764) -> (w763:string)
                                n519 = Two Button Dialog(message=w763, 1:w773, 2:w774) -> (T button?=w766:bool)
                                n520 = case shown="True" w766 {
                                tunnel: w772 -> [w777 w778]
                                tunnel: [w777 w778] -> w771
                                tunnel: [w776 w779] -> w770
                                tunnel: [w775 w779] -> w769
                                frame False {
                                n521 = Unbundle(w777) -> ("CYCLE"=w776:dbl, "MINS"=w775:dbl)  [unwired: 1 out]
                                }
                                frame True {
                                w779 = 0.0
                                }
                                }
                                n522 = Bundle(cluster=w771, "CYCLE"=w770, "MINS"=w769, "STATUS"="RUN") -> (w768:T4)
                                n523 = local write "DISP LAB01-1"(w768) -> ()
                              }
                              frame #4 {
                                n524 = local read "TEMP START LAB01-1"() -> (w782:cluster{"TL":dbl, "TN":dbl})
                                n525 = Bundle(cluster=w782, "TL"=w780, "TN"=w780) -> (w781:cluster{"TL":dbl, "TN":dbl})
                                n526 = local write "TEMP START LAB01-1"(w781) -> ()
                              }
                            }
                          }
                        }
                      }
                    }
                  }
                }
              }
              event "RUN LAB01-2": Value Change {
                n527 = event-data() -> ("NewVal"=w787:bool)  [unwired: 1 in, 5 out]
                n528 = local write "run lab01-2"(w787) -> ()
                n529 = case shown="True" w787 {
                  tunnel: w793 -> [_ w831]
                  tunnel: w792 -> [_ w830]
                  tunnel: w790 -> [w795 w829]
                  tunnel: w791 -> [_ w828]
                  tunnel: w789 -> [_ w827]
                  tunnel: [w794 w826] -> w788
                  tunnel: w786 -> [_ w825]
                  tunnel: w785 -> [_ w824]
                  tunnel: w784 -> [_ w823]
                  tunnel: w783 -> [_ w821]
                  frame False {
                    # "stop test"
                    n530 = stacked-sequence {
                      tunnel: w795 -> [w804 _]
                      tunnel: [w796 _] -> w794
                      frame #0 {
                        n531 = local read "DISP LAB01-2"() -> (w803:T4)
                        n532 = Unbundle(w803) -> ("CYCLE"=w801:dbl, "MINS"=w802:dbl)  [unwired: 1 out]
                        n533 = case shown="\"CHART TEST\", Default" w804 {
                          tunnel: w802 -> [_ _ w811]
                          tunnel: w801 -> [w809 w810 _]
                          tunnel: [w809 w810 w811] -> w800
                          frame "CHART TEST", Default {
                          }
                          frame "CYCLE TEST" {
                          }
                          frame "T-RISE TEST" {
                          }
                        }
                        n534 = local read "TDMS LAB01-2"() -> (w808:refnum<k34>)
                        n535 = Build Array("STOPPED") -> (w805:string[])
                        n536 = Build Array(w800) -> (w799:dbl[])
                        n537 = TDMS Write(0:w808, 5:"TEST RESULT", 7:w805, 9:w799) -> (4:w797:refnum<k34>, 15:w798:errorcluster)  [unwired: 2 in, 2 out]
                        n538 = TDMS Close(8:w798, 11:w797) -> (0:w796:errorcluster)  [unwired: 1 out]
                      }
                      frame #1 {
                        n539 = local read "DISP LAB01-2"() -> (w815:T4)
                        n540 = stacked-sequence {
                          tunnel: "LAB01-2" -> [w817 w819]
                          frame #0 {
                            n541 = call "sub vi - defrag tdms v1.vi"("panel id"=w817) -> ("error out"=w816:errorcluster)  [unwired: 10 in]
                            n542 = local write "data file error"(w816) -> ()
                          }
                          frame #1 {
                            n543 = call "Save data file (stop) v3.vi"("panel id"=w819) -> ("network file save error"=w818:errorcluster)  [unwired: 9 in, 1 out]
                            n544 = local write "RESULT LAB01-2"(FALSE) -> ()
                            n545 = local write "data file error"(w818) -> ()
                          }
                        }
                        n546 = Bundle(cluster=w815, "STATUS"="STOP") -> (w813:T4)  [unwired: 2 in]
                        n547 = local write "DISP LAB01-2"(w813) -> ()
                      }
                    }
                  }
                  frame True {
                    n548 = local read "SIG LAB01-2"() -> (w822:T2)
                    n549 = stacked-sequence {
                      seq-local: [w833 _] -> [_ w837]
                      tunnel: w831 -> [_ w847]
                      tunnel: w830 -> [_ w846]
                      tunnel: w829 -> [_ w845]
                      tunnel: w828 -> [_ w844]
                      tunnel: w827 -> [_ w843]
                      tunnel: [_ w842] -> w826
                      tunnel: w825 -> [_ w841]
                      tunnel: w824 -> [_ w840]
                      tunnel: w823 -> [_ w839]
                      tunnel: w822 -> [w832 w838]
                      tunnel: w821 -> [_ w836]
                      frame #0 {
                        n550 = Unbundle(w832) -> ("AMPS"=w835:dbl)  [unwired: 4 out]
                        n551 = call "Check For Amps on v1.vi"("ID"="LAB01-2", "amps"=w835) -> ("amps"=w833:bool)  [unwired: 9 in]
                      }
                      frame #1 {
                        n552 = case shown="True" w837 {
                          tunnel: w847 -> [_ w860]
                          tunnel: w846 -> [_ w859]
                          tunnel: w845 -> [_ w858]
                          tunnel: w844 -> [_ w857]
                          tunnel: w843 -> [_ w856]
                          tunnel: [errorcluster {"status"=FALSE, "code"=0, "source"=""} ("error out") w855] -> w842
                          tunnel: w841 -> [_ w854]
                          tunnel: w840 -> [_ w853]
                          tunnel: w839 -> [_ w852]
                          tunnel: w838 -> [_ w851]
                          tunnel: w836 -> [_ w850]
                          frame False {
                            w848 = FALSE
                            n553 = local write "RUN LAB01-2"(w848) -> ()
                            n554 = local write "run lab01-2"(w848) -> ()
                          }
                          frame True {
                            n555 = stacked-sequence {
                              seq-local: [w861 _ _ _ _] -> [_ w885 _ _ _]
                              tunnel: w860 -> [w866 _ _ _ _]
                              tunnel: w859 -> [w863 _ _ _ _]
                              tunnel: w858 -> [w876 _ _ _ _]
                              tunnel: w857 -> [w869 _ _ _ _]
                              tunnel: w856 -> [w864 _ _ _ _]
                              tunnel: [_ w880 _ _ _] -> w855
                              tunnel: w854 -> [_ _ _ w907 _]
                              tunnel: w853 -> [_ _ _ w906 _]
                              tunnel: w852 -> [_ _ _ w905 _]
                              tunnel: w851 -> [_ _ _ _ _]
                              tunnel: w850 -> [_ _ _ _ w920]
                              frame #0 {
                                w862 = "\\"
                                n556 = local read "SET LAB01-2"() -> (w871:T5)
                                n557 = case shown="\"CYCLE TEST\"" w876 {
                                tunnel: ["L01-2-CHART TEST-" "L01-2-CYCLE TEST-" "L01-2-T-RISE TEST-"] -> w872
                                frame "CHART TEST", Default {
                                }
                                frame "CYCLE TEST" {
                                }
                                frame "T-RISE TEST" {
                                }
                                }
                                n558 = Unbundle(w871) -> ("DESCRIPTION"=w870:string)  [unwired: 4 out]
                                n559 = Concatenate Strings(w866, "\\", w864, w862, w863, w862) -> (w873:string)
                                n560 = String To Path(string=w873) -> (path=w875:path)
                                n561 = Concatenate Strings(w873, w872, w870, "-", w869, ".tdms") -> (w861:string)
                                n562 = Create Folder(path (use dialog)=w875) -> (error out=w874:errorcluster)  [unwired: 2 in, 2 out]
                                n563 = call <vilib>:"Clear Errors.vi"("error in (no error)"=w874) -> ()  [unwired: 6 in, 1 out]
                                n564 = global write "Global 1.vi" "LAB01-2 FILE"(w861) -> ()
                              }
                              frame #1 {
                                (unwired) FALSE
                                n565 = String To Path(string=w885) -> (path=w881:path)
                                n566 = TDMS Open(6:FALSE, 10:T20."create or replace" ("operation (0:open)"), 11:w881) -> (0:w880:errorcluster, 3:→"TDMS LAB01-2":refnum<k34>)  [unwired: 4 in]
                              }
                              frame #2 {
                                n567 = local read "SET LAB01-2"() -> (w891:T5)
                                n568 = local read "TDMS LAB01-2"() -> (w902:refnum<k34>)
